vi "StartAOVoltage.vi"(0 "Physical Channel(s)":tag="DAQ/ao0", 5 "Max Voltage":dbl=10.0, 7 "Min Voltage":dbl=-10.0, 9 "Parameters":T1={"Waveform Type"=0, "Desired Frequency"=1000.0, "Amplitude"=1.0, "Offset"=0.0, "Samples per Buffer"=8000.0, "Cycles per Buffer"=250} {"Waveform Type" items=[" Sine Wave", " Triangle Wave", " Square Wave", " Sawtooth Wave"]}) -> (15 "error out":errorcluster)   [LabVIEW 2012]
doc: "I. Description:\nThis example demonstrates how to continuously output a waveform using an internal sample clock. The output waveform will be stored on the on-board memory of the device and then generated continuously from there.\n\nII. Instructions for Running:\n1. Select the Physical Channel to correspond to where your signal is output on the DAQ device.\n2. Enter the Minimum and Maximum Voltage Ranges.\n3. Specify the Desired Frequency of the output Waveform\n4. Enter the Waveform Information. See the documentation of the Waveform Buffer Generation SubVI for information on each parameter.\nNOTE: Make sure the total number of samples contained in the Analog Output Waveform does not exceed the size of the on-board memory of the device.\n\n\nIII. Block Diagram Steps:\n1. Create an Analog Output Voltage Task\n2. Call the DAQmx Timing (Use Waveform) VI which sets the sample clock rate based on the input waveform parameters, and set the sample mode to Continuous.\n3. Configure the analog output operation to store the waveform on the on-board memory of the device.\n4. Write the waveform to the output buffer.\n5. Call the Start VI.\n6. Loop continuously until the user presses the Stop button. Check for errors every 100 ms using the Is Task Done? VI\n7. Call the Clear Task VI to clear the Task.\n8. Use the popup dialog box to display an error or warning if any.\n\nIV. I/O Connections Overview:\nMake sure your signal output terminal matches the Physical Channel I/O Control. For further connection information, refer to your hardware reference manual."
uses:
  <vilib>/DAQmx/write.llb/DAQmx Write (Analog 1D Wfm NChan NSamp).vi
  <vilib>/DAQmx/create/channels.llb/DAQmx Create Channel (AO-Voltage-Basic).vi
  <vilib>/DAQmx/configure/timing.llb/DAQmx Timing (Use Waveform).vi
  <vilib>/DAQmx/miscellaneous.llb/DAQmx Fill In Error Info.vi
  <resource>/objmgr/daqmx.rc
panel:
  out "Sample Rate":dbl
  out "dt":dbl
  out "Output Waveforms":waveform(dbl)[](graph) caption="Output Waveform"
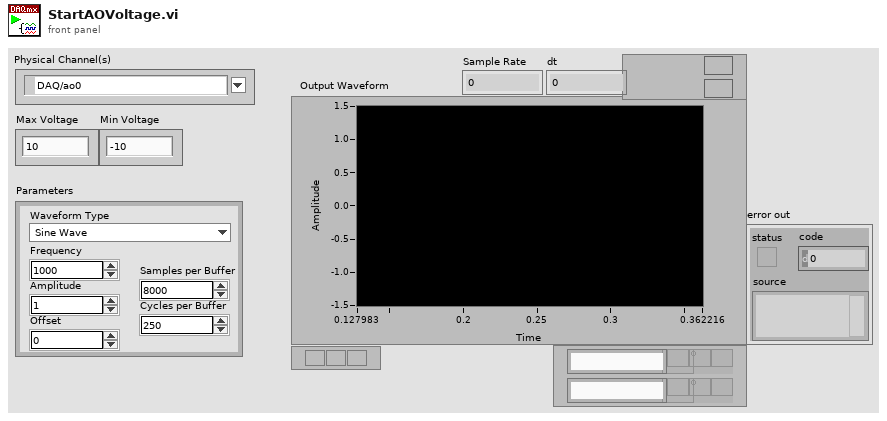
[diagram p1: front panel]
types:
  T1 = cluster{"Waveform Type":u16, "Desired Frequency":dbl, "Amplitude":dbl, "Offset":dbl, "Samples per Buffer":dbl, "Cycles per Buffer":i32}
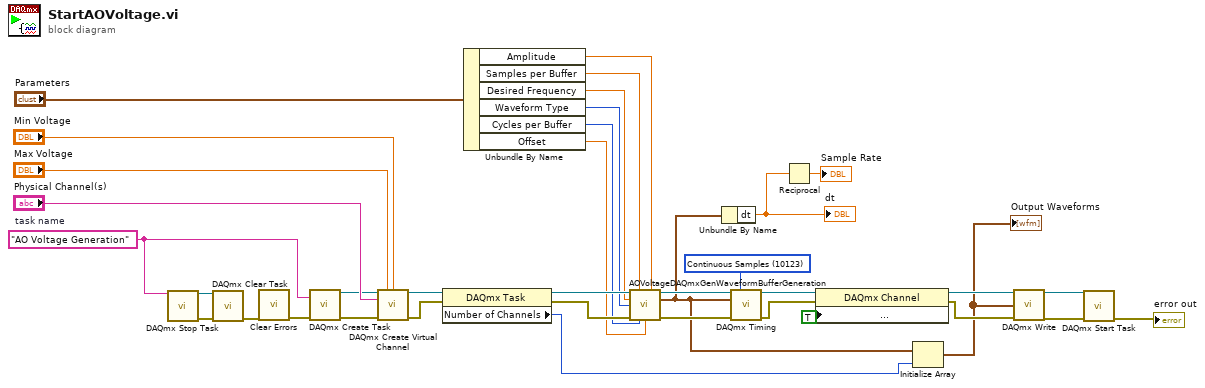
[diagram p0: block diagram]
diagram:
  w6 = "AO Voltage Generation"  # task name
  w18 = 10123 items=["Finite Samples"=10178, "Continuous Samples"=10123] ("sample mode")
  n1 = call <vilib>:"DAQmx Stop Task.vi"("task/channels in"=w6) -> ("task out"=w8:refnum<k21>, "error out"=w7:errorcluster)  [unwired: 13 in]
  n2 = call <vilib>:"DAQmx Clear Task.vi"("task in"=w8, "error in"=w7) -> ("error out"=w5:errorcluster)  [unwired: 13 in]
  n3 = call <vilib>:"Clear Errors.vi"("error in (no error)"=w5) -> ("error out"=w4:errorcluster)  [unwired: 6 in]
  n4 = call <vilib>:"DAQmx Create Task.vi"("new task name"=w6, "error in"=w4) -> ("task out"=w9:refnum<k21>, "error out"=w10:errorcluster)  [unwired: 12 in]
  n5 = call-poly <vilib>:"DAQmx Create Virtual Channel.vi"("task in"=w9, "maximum value"="Max Voltage", "minimum value"="Min Voltage", "physical channels"="Physical Channel(s)", "error in"=w10) -> ("task out"=w11:refnum<k21>, "error out"=w22:errorcluster)  [unwired: 9 in]
  n6 = property class="DAQmx Task"(reference=w11, error in=w22) -> (reference out=w34:refnum<k21>, error out=w33:errorcluster, "Number of Channels"=w15:u32)
  n7 = Unbundle By Name("Parameters") -> ("Amplitude"=w31:dbl, "Samples per Buffer"=w30:dbl, "Desired Frequency"=w29:dbl, "Waveform Type"=w28:u16, "Cycles per Buffer"=w27:i32, "Offset"=w26:dbl)
  n8 = call "AOVoltageDAQmxGenWaveformBufferGeneration.vi"("task/channels in"=w34, "Samples per Buffer"=w30, "Amplitude"=w31, "Desired Frequency"=w29, "Waveform Type"=w28, "error in (no error)"=w33, "Cycles per Buffer"=w27, "Offset"=w26) -> ("task out"=w16:refnum<k21>, "Waveform"=w3:waveform(dbl), "error out"=w17:errorcluster)  [unwired: 3 in, 2 out]
  n9 = Unbundle By Name(w3) -> ("dt"=w2:dbl)
  "dt" <- w2
  n10 = call-poly <vilib>:"DAQmx Timing.vi"("task/channels in"=w16, "sample mode"=w18, "waveform"=w3, "error in"=w17) -> ("task out"=w20:refnum<k21>, "error out"=w21:errorcluster)  [unwired: 10 in]
  n11 = Reciprocal(x=w2) -> (1/x=→"Sample Rate":dbl)
  n12 = property class="DAQmx Channel"(reference=w20, error in=w21, "Analog Output:General Properties:Advanced:Data Transfer and Memory:Use Only Onboard Memory"=TRUE ("AO.UseOnlyOnBrdMem")) -> (reference out=w14:refnum<k21>, error out=w35:errorcluster)
  n13 = Initialize Array(w3, w15) -> (w13:waveform(dbl)[])
  "Output Waveforms" <- w13
  n14 = call-poly <vilib>:"DAQmx Write.vi"("task/channels in"=w14, "data"=w13, "error in"=w35) -> ("task out"=w37:refnum<k21>, "error out"=w36:errorcluster)  [unwired: 10 in, 1 out]
  n15 = call <vilib>:"DAQmx Start Task.vi"("task/channels in"=w37, "error in"=w36) -> ("error out"=→"error out":errorcluster)  [unwired: 12 in, 1 out]
